vi "Message - Password.vi"(8 "error in":errorcluster) -> (0 "error out":errorcluster, 3 "Right Info?":bool)   [LabVIEW 2014]
panel:
  in  "PASSWORD":string
  in  "USERNAME":string
  out "Warning":u16(ring)
  in  "Cancel":bool
  in  "Login":bool
  # "LOGIN INFORMATION"
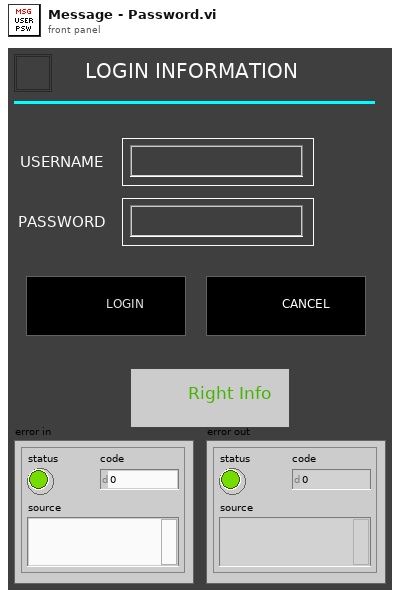
[diagram p1: front panel]
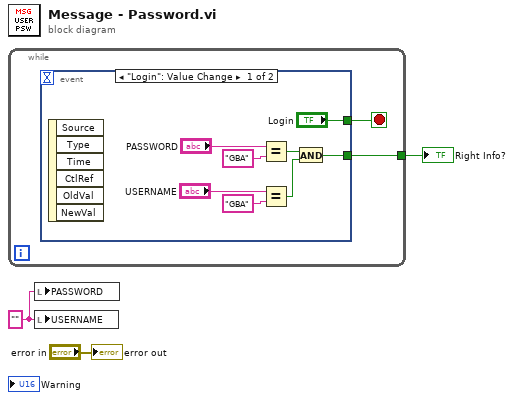
[diagram p0: block diagram]
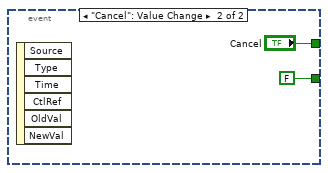
[diagram p2: hidden frame]
diagram:
  w1 = "" ("PASSWROD")
  n1 = while {
    tunnel: [w5] -> w3
    stop <- w4 stop-if-true
    n2 = event shown="[0] \"Login\": Value Change" {
      selector: _ -> [_ _]
      dyn-events: _ -> [_ _]
      timeout: _ -> [_ _]
      tunnel: ["Login" "Cancel"] -> w4
      tunnel: [w6 FALSE ("YES Button")] -> w5
      event "Login": Value Change {
        n3 = event-data() -> ()  [unwired: 1 in, 6 out]
        n4 = Equal?(x="PASSWORD", y="GBA") -> (x = y?=w8:bool)
        n5 = Equal?(x="USERNAME", y="GBA") -> (x = y?=w7:bool)
        n6 = And(x=w8, y=w7) -> (x .and. y?=w6:bool)
      }
      event "Cancel": Value Change {
        n7 = event-data() -> ()  [unwired: 1 in, 6 out]
      }
    }
  }
  "Right Info?" <- w3
  n8 = local write "PASSWORD"(w1) -> ()
  n9 = local write "USERNAME"(w1) -> ()
  "error out" <- "error in"
